vi "Fetch Multi Eval Meas List ACLR NR Carrier Frequency Results.vi"(6 "Carrier Frequency (Positive)":i32(ring)=1 items=["Negative", "Positive"], 8 "error in (no error)":errorcluster, 9 "Result Type (Current)":i32(ring) items=["Current", "Average"], 10 "Instance (1)":T1=1, 11 "VISA resource name":refnum<visa-resource-name>) -> (0 "error out":errorcluster, 1 "Results":dbl[](array[numeric]) format="%^.3e", 2 "Reliability":i32, 3 "VISA resource name out":refnum<visa-resource-name>)   [LabVIEW 2020, in "Rohde&Schwarz CMWXP NR FR1 Measurement.lvlib"]
doc: "Return the ACLR for the first adjacent NR channel above (Positive) or below (Negative) the carrier frequency for all measured list mode segments.\n\nAttributes:\nRSCMWXPNRFR1M_ATTR_FETCH_MULTI_EVAL_MEAS_LIST_ACLR_NR_NEGATIVE_CURRENT_RESULTS\nRSCMWXPNRFR1M_ATTR_FETCH_MULTI_EVAL_MEAS_LIST_ACLR_NR_NEGATIVE_AVERAGE_RESULTS\nRSCMWXPNRFR1M_ATTR_FETCH_MULTI_EVAL_MEAS_LIST_ACLR_NR_POSITIVE_CURRENT_RESULTS\nRSCMWXPNRFR1M_ATTR_FETCH_MULTI_EVAL_MEAS_LIST_ACLR_NR_POSITIVE_AVERAGE_RESULTS\n\nRemote-control commands:\nFETCh:NRSub:MEAS<i>:MEValuation:LIST:ACLR:NR:NEGativ:CURRent?\nFETCh:NRSub:MEAS<i>:MEValuation:LIST:ACLR:NR:NEGativ:AVERage?\nFETCh:NRSub:MEAS<i>:MEValuation:LIST:ACLR:NR:POSitiv:CURRent?\nFETCh:NRSub:MEAS<i>:MEValuation:LIST:ACLR:NR:POSitiv:AVERage?"
uses:
  <instrlib>/Rohde&Schwarz CMWXP NR FR1 Measurement/Rohde&Schwarz CMWXP NR FR1 Measurement.lvlib
  <instrlib>/Rohde&Schwarz CMWXP NR FR1 Measurement/Private/_Instance.ctl
  <instrlib>/Rohde&Schwarz CMWXP NR FR1 Measurement/Private/rsidr_core.llb/rsidr_core.lvlib
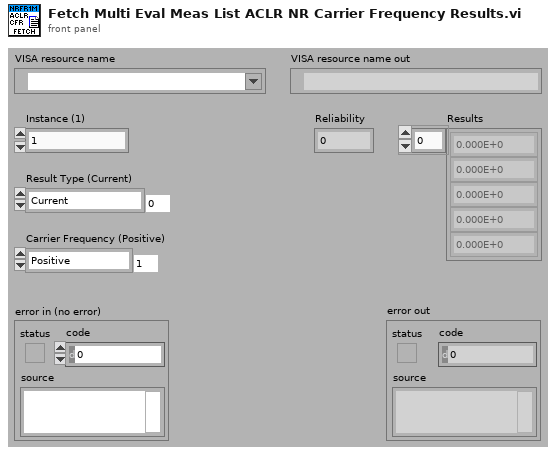
[diagram p1: front panel]
types:
  T1 = typedef "Rohde&Schwarz CMWXP NR FR1 Measurement.lvlib/_Instance.ctl" = i32
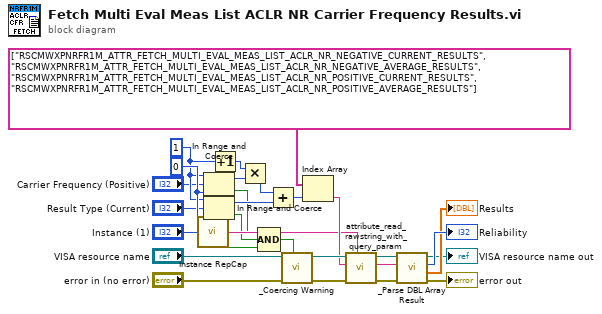
[diagram p0: block diagram]
diagram:
  w10 = 1
  w12 = 0
  n1 = call <instrlib>:"Instance RepCap.vi"("Instance In"="Instance (1)") -> ("In Range?"=w5:bool, "RepCap Identifier Out"=w21:string)  [unwired: 1 in]
  n2 = In Range and Coerce(upper limit=w10, x="Carrier Frequency (Positive)", lower limit=w12) -> (coerced(x)=w11:i32, In Range?=w3:bool)
  n3 = In Range and Coerce(upper limit=w10, x="Result Type (Current)", lower limit=w12) -> (coerced(x)=w13:i32, In Range?=w4:bool)
  n4 = Increment(x=w10) -> (x+1=w9:i32)
  n5 = Multiply(x=w9, y=w11) -> (x*y=w8:i32)
  n6 = Compound Arithmetic op=AND(w3, w4, w5) -> (w2:bool)
  n7 = Add(x=w8, y=w13) -> (x+y=w1:i32)
  n8 = call <instrlib>:"_Coercing Warning.vi"("In Range?"=w2, "error in (no error)"="error in (no error)", "VISA resource name"="VISA resource name") -> ("error out"=w22:errorcluster, "VISA resource name out"=w24:refnum<visa-resource-name>)  [unwired: 7 in]
  n9 = Index Array(array=string[] ["RSCMWXPNRFR1M_ATTR_FETCH_MULTI_EVAL_MEAS_LIST_ACLR_NR_NEGATIVE_CURRENT_RESULTS", "RSCMWXPNRFR1M_ATTR_FETCH_MULTI_EVAL_MEAS_LIST_ACLR_NR_NEGATIVE_AVERAGE_RESULTS", "RSCMWXPNRFR1M_ATTR_FETCH_MULTI_EVAL_MEAS_LIST_ACLR_NR_POSITIVE_CURRENT_RESULTS", "RSCMWXPNRFR1M_ATTR_FETCH_MULTI_EVAL_MEAS_LIST_ACLR_NR_POSITIVE_AVERAGE_RESULTS"], index=w1) -> (element=w23:string)
  n10 = call <instrlib>:"attribute_read_rawstring_with_query_param.vi"("Repeated Capability"=w21, "error in"=w22, "Attribute ID"=w23, "VISA resource name"=w24) -> ("error out"=w20:errorcluster, "Raw String out"=w19:string, "VISA resource name out"=w18:refnum<visa-resource-name>)  [unwired: 5 in]
  n11 = call <instrlib>:"_Parse DBL Array Result.vi"("error in (no error)"=w20, "Input String"=w19, "VISA resource name"=w18) -> ("error out"=→"error out":errorcluster, "Results"=→"Results":dbl[], "Reliability"=→"Reliability":i32, "VISA resource name out"=→"VISA resource name out":refnum<visa-resource-name>)  [unwired: 5 in]
